vi "test picture to arr.vi"() -> ()   [LabVIEW 2018, in "LV-Julia_ZMQ-Roundtrip_lib.lvlib"]
uses:
  LV-Julia_ZMQ-Roundtrip_lib.lvlib
  Bindata description.ctl
  <vilib>/picture/picture.llb/imagedata.ctl
  997e3e12-d239-4053-9461-1027462df242.vi
  997e3e12-d239-4053-9461-1027462df242.vi/9937c24d-da9a-4863-ac90-ba40682b48ca.vi
  997e3e12-d239-4053-9461-1027462df242.vi/9937c24d-da9a-4863-ac90-ba40682b48ca.vi/59b608c6-7562-4867-8403-c3e07949bd6d.vi
  check ID validity.vi
  <vilib>/Utility/error.llb/Error Cluster From Error Code.vi
panel:
  out "image data":T1
  out "new picture 2":picture
  out "Bindata & descr out":cluster{"bindata_descr":T2[], "bindata":u8[]}
  out "error out":errorcluster
  out "new picture":picture
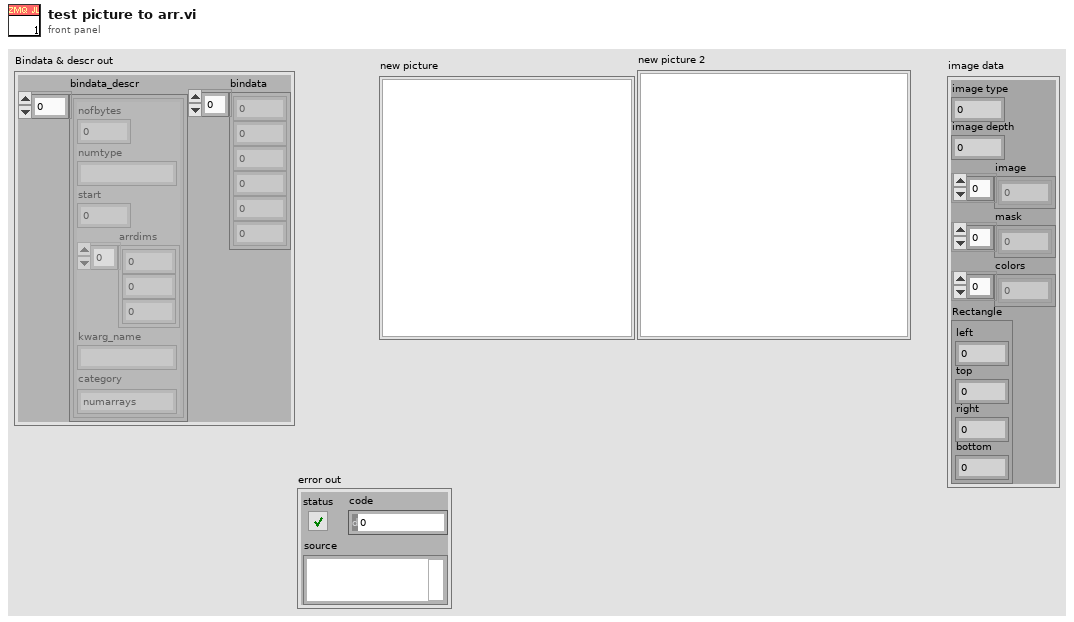
[diagram p1: front panel]
types:
  T1 = typedef "imagedata.ctl" = cluster{"image type":i32, "image depth":i32, "image":u8[], "mask":u8[], "colors":u32[], "Rectangle":cluster{"left":i16, "top":i16, "right":i16, "bottom":i16}}
  T2 = typedef "LV-Julia_ZMQ-Roundtrip_lib.lvlib/Bindata description.ctl" = cluster{"nofbytes":i32, "numtype":string, "start":i32, "arrdims":i32[], "kwarg_name":string, "category":string}
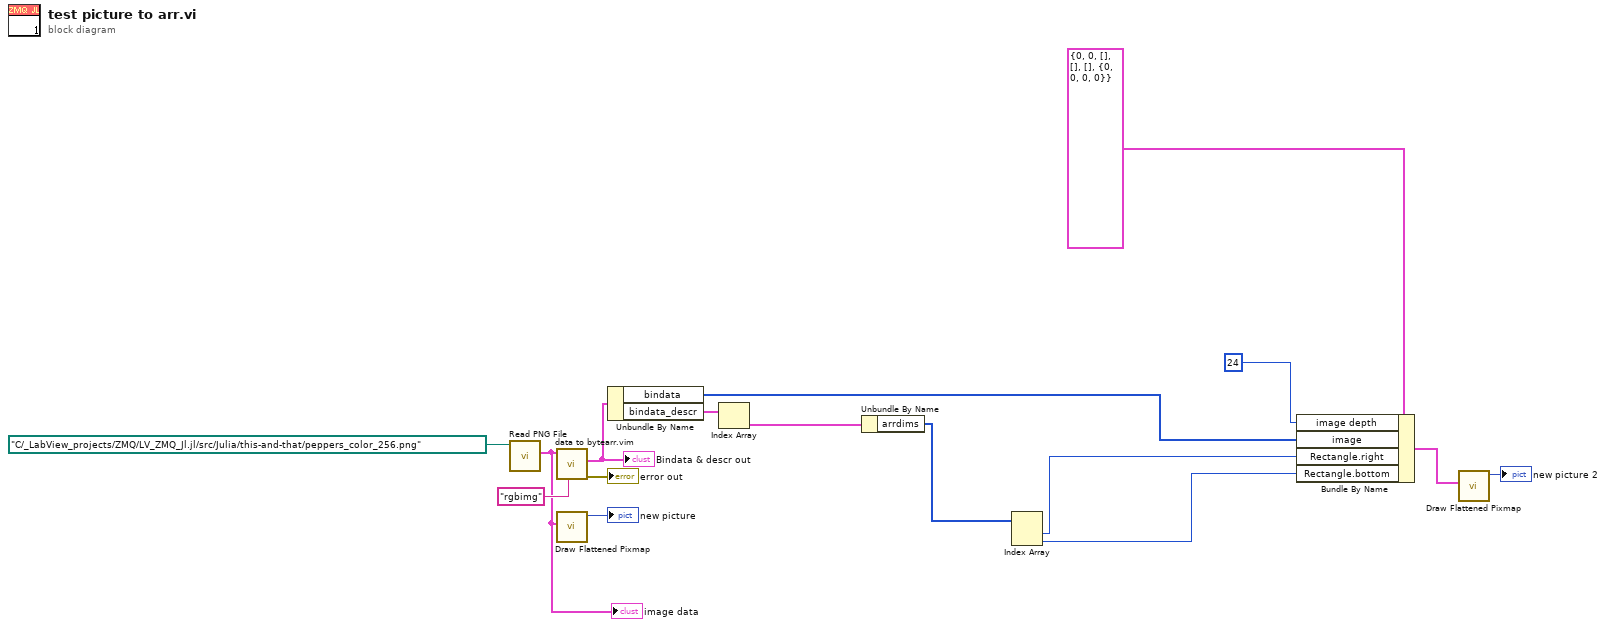
[diagram p0: block diagram]
diagram:
  n1 = call <vilib>:"Read PNG File.vi"("path to PNG file"=path "C:/_LabView_projects/ZMQ/LV_ZMQ_Jl.jl/src/Julia/this-and-that/peppers_color_256.png" ("Path")) -> ("image data"=w8:T1)  [unwired: 8 in, 2 out]
  "image data" <- w8
  n2 = call "data to bytearr.vim"("kwarg_name"="rgbimg" ("Tag"), "data in"=w8) -> ("error out"=→"error out":errorcluster, "Bindata & descr out"=w12:cluster{"bindata_descr":T2[], "bindata":u8[]})  [unwired: 7 in, 1 out]
  "Bindata & descr out" <- w12
  n3 = call <vilib>:"Draw Flattened Pixmap.vi"("image data"=w8) -> ("new picture"=→"new picture":picture)  [unwired: 8 in]
  n4 = Unbundle By Name(w12) -> ("bindata"=w4:u8[], "bindata_descr"=w11:T2[])
  n5 = Index Array(array=w11) -> (element=w10:T2)  [unwired: 1 in]
  n6 = Unbundle By Name(w10) -> ("arrdims"=w3:i32[])
  n7 = Index Array(array=w3) -> (element #1=w2:i32, element #2=w1:i32)  [unwired: 2 in]
  n8 = Bundle By Name(cluster=T1 {"image type"=0, "image depth"=0, "image"=[], "mask"=[], "colors"=[], "Rectangle"={"left"=0, "top"=0, "right"=0, "bottom"=0}} ("image data"), "image depth"=24, "image"=w4, "Rectangle.right"=w2, "Rectangle.bottom"=w1) -> (w6:T1)
  n9 = call <vilib>:"Draw Flattened Pixmap.vi"("image data"=w6) -> ("new picture"=→"new picture 2":picture)  [unwired: 8 in]
